vi "Trim and Filter Bead (SubVI).vi"(8 "Saturation":dbl=5.0, 9 "Target Length":dbl, 10 "Start OFFSET":dbl, 11 "Raw Scan Data":dbl[][](array[numeric])) -> (3 "Filtered Bead":cluster{dbl[], dbl[]})   [LabVIEW 2016]
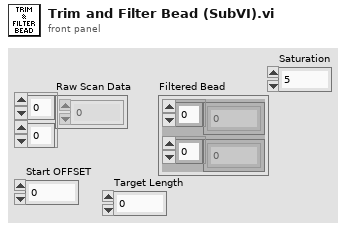
[diagram p1: front panel]
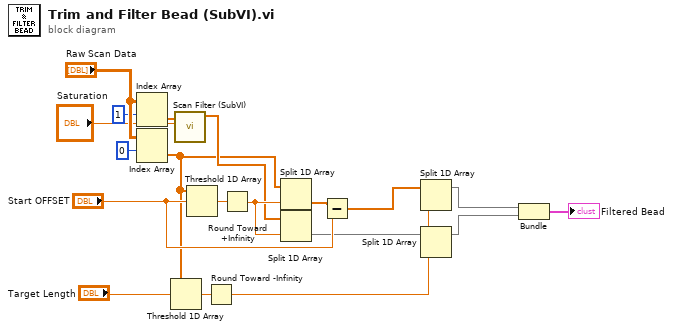
[diagram p0: block diagram]
diagram:
  n1 = Index Array(array="Raw Scan Data", index (row)=1) -> (element=w16:dbl[])  [unwired: 1 in]
  n2 = Index Array(array="Raw Scan Data", index (row)=0) -> (element=w8:dbl[])  [unwired: 1 in]
  n3 = Threshold 1D Array(2:"Target Length", 3:w8) -> (0:w9:dbl)  [unwired: 1 in]
  n4 = call "Scan Filter (SubVI).vi"("Saturation"="Saturation", "Array in"=w16) -> ("Array out"=w18:dbl[])  [unwired: 9 in]
  n5 = Threshold 1D Array(2:"Start OFFSET", 3:w8) -> (0:w17:dbl)  [unwired: 1 in]
  n6 = Round Toward -Infinity(1:w9) -> (0:w5:dbl)
  n7 = Round Toward +Infinity(x=w17) -> (ceil(x): smallest int >= x=w19:dbl)
  n8 = Split 1D Array(array=w8, index=w19) -> (second subarray=w12:dbl[])  [unwired: 1 out]
  n9 = Split 1D Array(array=w18, index=w19) -> (second subarray=w4:dbl[])  [unwired: 1 out]
  n10 = Subtract(x=w12, y="Start OFFSET") -> (x-y=w7:dbl[])
  n11 = Split 1D Array(array=w7, index=w5) -> (first subarray=w6:dbl[])  [unwired: 1 out]
  n12 = Split 1D Array(array=w4, index=w5) -> (first subarray=w3:dbl[])  [unwired: 1 out]
  n13 = Bundle(w6, w3) -> (→"Filtered Bead":cluster{dbl[], dbl[]})  [unwired: 1 in]
